vi "Teleop.vi"(10 "Match Info":T1={"Autonomous Elapsed Seconds"=0.0, "TeleOp Elapsed Seconds"=0.0, "Disabled Elapsed Seconds"=0.0, "Visited Autonomous"=FALSE, "Visited TeleOp"=FALSE, "Visited Disabled"=FALSE, "Autonomous Settings"={"Autonomous Style"=enum."Independent", "VI Refnum"=refnum}}, 11 "Call Context":T2) -> ()   [LabVIEW 2013]
doc: "This VI is called for each TeleOp packet received from the DS where the robot is not disabled. It is often used to read from the joysticks and update I/O or to update setpoints for timed control loops. It should complete and return within 20 milliseconds or it may miss DS packets."
uses:
  <vilib>/Rock Robotics/WPI/DriverStation/WPI_DriverStationDerivedRobotMode.ctl
  <vilib>/Rock Robotics/WPI/DriverStation/WPI_DriverStationMatch Info.ctl
  Robot Global Data.vi
  <vilib>/Rock Robotics/WPI/Joystick/WPI_JoystickGetSetRefNum.vi
  <vilib>/Rock Robotics/WPI/RobotDrive/WPI_RobotDriveGetSetRefNum.vi
  <vilib>/Rock Robotics/WPI/RobotDrive/WPI_RobotDriveArcadeDrive_Standard(NoSaturation).vi
panel:
  out "Yaxis 2":dbl
  in  "YAxis":dbl
  in  "StockArcade?":bool
  in  "Ramp?":bool=TRUE
  in  "Yaxis":dbl
  in  "Mult":dbl=0.0010912021824043647
  in  "x":dbl=1.1
  in  "y":dbl=0.95
  out "Numeric 1":dbl(slide) scale=0.0..100.0
  out "Boolean 2":bool
  out "Boolean 1":bool
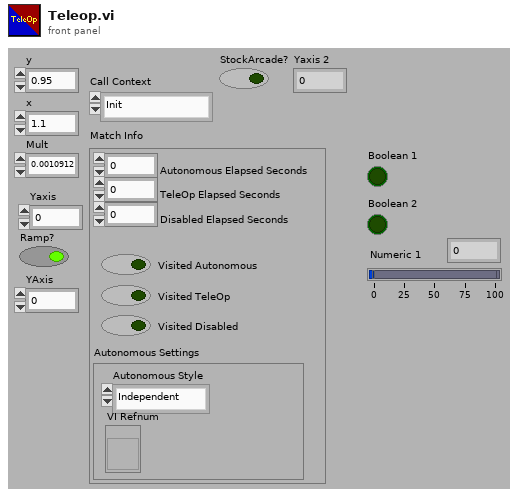
[diagram p1: front panel]
types:
  T1 = typedef "WPI_DriverStationMatch Info.ctl" = cluster{"Autonomous Elapsed Seconds":dbl, "TeleOp Elapsed Seconds":dbl, "Disabled Elapsed Seconds":dbl, "Visited Autonomous":bool, "Visited TeleOp":bool, "Visited Disabled":bool, "Autonomous Settings":cluster{"Autonomous Style":enum16{"Iterative", "Independent"}, "VI Refnum":refnum<vi>}}
  T2 = typedef "WPI_DriverStationDerivedRobotMode.ctl" = enum16{"Init", "Execute", "Stop"}
  T3 = typedef "WPI_JoystickDevRef.ctl" = cluster{"Device":T4}
  T4 = typedef "WPI_JoystickDeviceEnum.ctl" = enum16{"USB 1", "USB 2", "USB 3", "USB 4", "Kinect 1", "Kinect 2"}
  T5 = cluster{"axis 1 (x)":dbl, "axis 2 (y)":dbl, "axis 3 (throttle)":dbl, "axis 4":dbl, "axis 5":dbl, "axis 6":dbl}
  T6 = typedef "WPI_JoystickButtonState.ctl" = cluster{"Button 1":bool, "Button 2":bool, "Button 3":bool, "Button 4":bool, "Button 5":bool, "Button 6":bool, "Button 7":bool, "Button 8":bool, "Button 9":bool, "Button 10":bool, "Button 11":bool, "Button 12":bool}
  T7 = typedef "WPI_MotorControlDeviceRef.ctl" = cluster{"DeviceStatus":errorcluster, "Type":enum16{"PWM", "CAN"}, "PWM":cluster{"Digital Module":T8, "PWM Channel":T9, "DeadBand":T10}, "CAN":cluster{"Device Number":u8, "Control Mode":T11, "Semaphore":T12, "Max Vout":dbl}, "Invert":bool, "TransformRef":T13, "InvTransformRef":T13}
  T8 = typedef "FPGA_TypedefDigitalModule.ctl" = enum16{"Digital Module 1", "Digital Module 2"}
  T9 = typedef "FPGA_DIOPWMChannel.ctl" = enum8{"PWM 1", "PWM 2", "PWM 3", "PWM 4", "PWM 5", "PWM 6", "PWM 7", "PWM 8", "PWM 9", "PWM 10", "Invalid"}
  T10 = typedef "WPI_PWMDeadband.ctl" = cluster{"Name":string, "maxPositivePwm":i32, "minPositivePwm":i32, "centerPwm":i32, "maxNegativePwm":i32, "minNegativePwm":i32, "angularRange":u16}
  T11 = typedef "WPI_CANJaguar_ControlMode.ctl" = enum8{"Percent VBus", "Current", "Speed", "Position", "Voltage"}
  T12 = typedef "Semaphore RefNum" = refnum<k1>
  T13 = typedef "WPI_PWMTransform_ConPane.ctl" = refnum<vi>
  T14 = typedef "WPI_RobotDriveDevRef.ctl" = cluster{"DevStatus":errorcluster, "Motors[]":T7[], "Square Inputs":bool, "Max Output":dbl, "Isochronous":bool}
  T15 = typedef "WPI_ServoDeviceRef.ctl" = cluster{"DeviceStatus":errorcluster, "Digital Module":T8, "PWM Channel":T9, "DeadBand":T10}
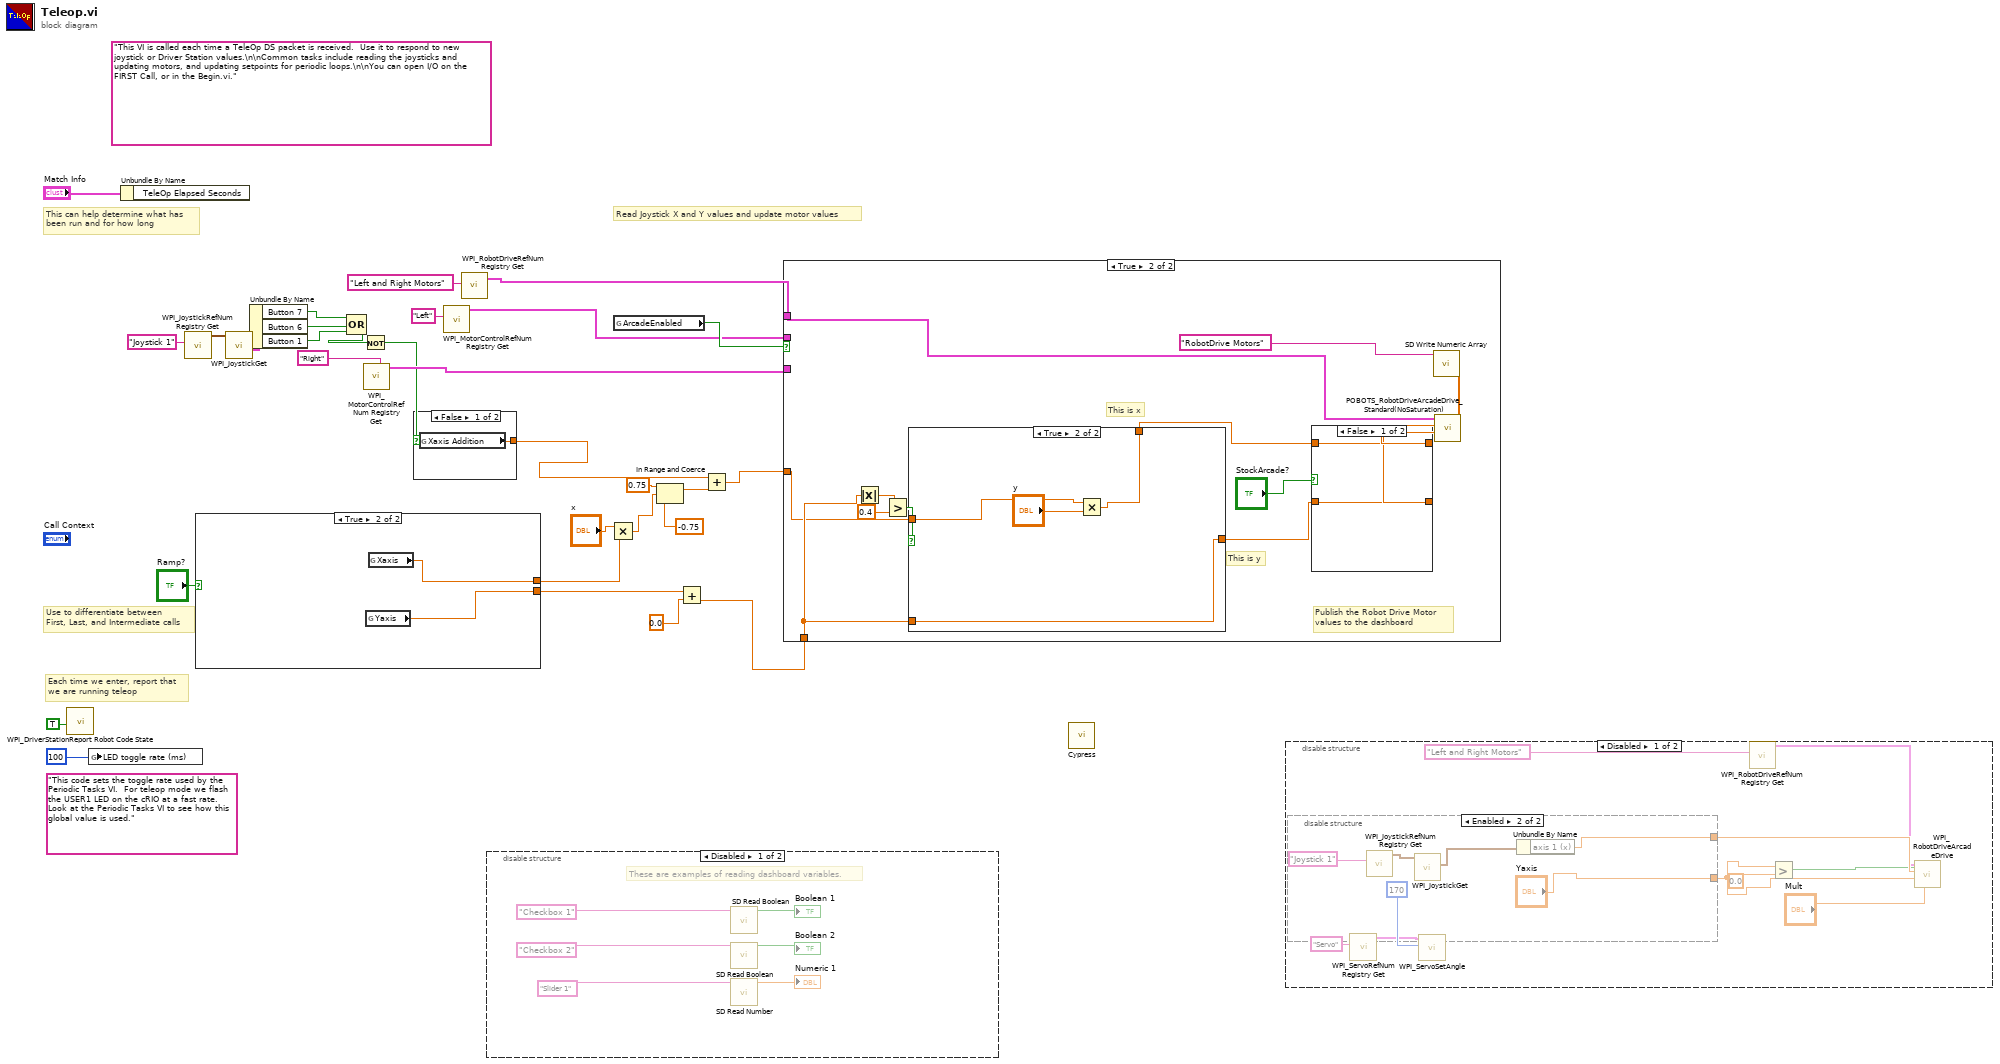
[diagram p0: block diagram]
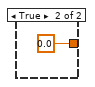
[diagram p2: hidden frame]
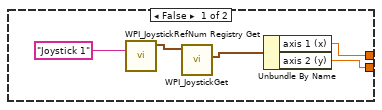
[diagram p3: hidden frame]
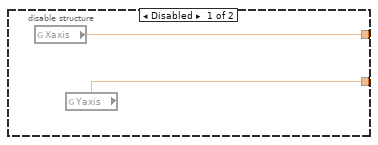
[diagram p4: hidden frame]
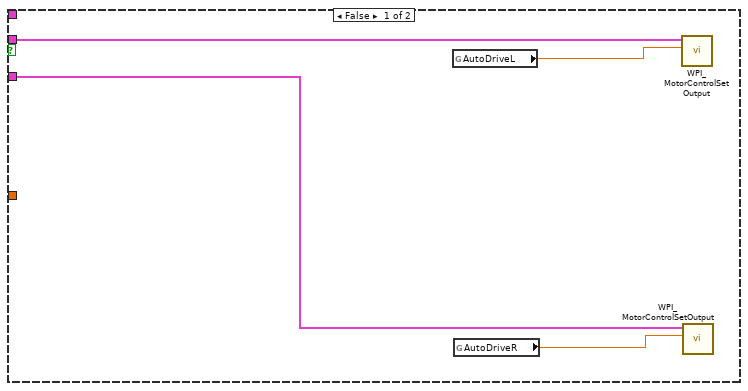
[diagram p6: hidden frame]
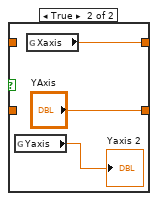
[diagram p7: hidden frame]
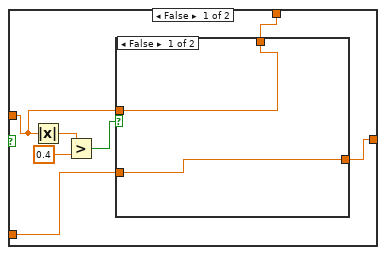
[diagram p8: hidden frame]
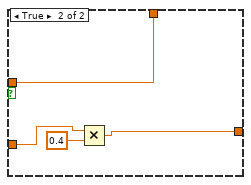
[diagram p9: hidden frame]
diagram:
  (unwired) "This code sets the toggle rate used by the Periodic Tasks VI.  For teleop mode we flash the USER1 LED on the cRIO at a fast rate.  Look at the Periodic Tasks VI to see how this global value is used."
  (unwired) "This VI is called each time a TeleOp DS packet is received.  Use it to respond to new joystick or Driver Station values.\n\nCommon tasks include reading the joysticks and updating motors, and updating setpoints for periodic loops.\n\nYou can open I/O on the FIRST Call, or in the Begin.vi."
  # "Publish the Robot Drive Motor\nvalues to the dashboard"
  # "Read Joystick X and Y values and update motor values"
  # "Each time we enter, report that\nwe are running teleop"
  # "Use to differentiate between\nFirst, Last, and Intermediate calls"
  # "This can help determine what has\nbeen run and for how long"
  n1 = call <vilib>:"WPI_DriverStationReport Robot Code State.vi"("TeleOp"=TRUE ("Autonomous")) -> ()  [unwired: 10 in, 1 out]
  n2 = global write "Robot Global Data.vi" "LED toggle rate (ms)"(u32 100 ("LED ms toggle rate")) -> ()
  n3 = Unbundle By Name("Match Info") -> ()  [unwired: 1 out]
  n4 = call <vilib>:"WPI_JoystickRefNum Registry Get.vi"("refnum name"="Joystick 1") -> ("JoystickDevRef"=w7:T3)  [unwired: 9 in, 1 out]
  n5 = case shown="True" "Ramp?" {
    tunnel: [w32 w37] -> w24
    tunnel: [w31 w36] -> w22
    frame False {
      n6 = call <vilib>:"WPI_JoystickRefNum Registry Get.vi"("refnum name"="Joystick 1") -> ("JoystickDevRef"=w34:T3)  [unwired: 9 in, 1 out]
      n7 = call <vilib>:"WPI_JoystickGet.vi"("JoystickDevRef"=w34) -> ("Axes"=w33:T5)  [unwired: 4 in, 2 out]
      n8 = Unbundle By Name(w33) -> ("axis 1 (x)"=w32:dbl, "axis 2 (y)"=w31:dbl)
    }
    frame True {
      n9 = global read "Robot Global Data.vi" "Yaxis"() -> (w36:dbl)
      n10 = global read "Robot Global Data.vi" "Xaxis"() -> (w37:dbl)
    }
  }
  n11 = call <vilib>:"WPI_JoystickGet.vi"("JoystickDevRef"=w7) -> ("Buttons"=w6:T6)  [unwired: 4 in, 2 out]
  n12 = Unbundle By Name(w6) -> ("Button 7"=w1:bool, "Button 6"=w2:bool, "Button 1"=w5:bool)
  n13 = Compound Arithmetic op=OR(w1, w2, w5) -> (w3:bool)
  n14 = Not(x=w3) -> (.not. x?=w4:bool)
  n15 = call <vilib>:"WPI_MotorControlRefNum Registry Get.vi"("refnum name"="Right") -> ("MotorControlDevRef"=w17:T7)  [unwired: 9 in, 1 out]
  n16 = case shown="False" w4 {
    tunnel: [w38 0.0 ("x")] -> w9
    frame False {
      n17 = global read "Robot Global Data.vi" "Xaxis Addition"() -> (w38:dbl)
    }
    frame True {
    }
  }
  n18 = call <vilib>:"WPI_MotorControlRefNum Registry Get.vi"("refnum name"="Left") -> ("MotorControlDevRef"=w18:T7)  [unwired: 9 in, 1 out]
  n19 = call <vilib>:"WPI_RobotDriveRefNum Registry Get.vi"("refnum name"="Left and Right Motors") -> ("RobotDriveDevRef"=w27:T14)  [unwired: 9 in, 1 out]
  n20 = disable-structure shown="Disabled" {
    frame Disabled {
      # "These are examples of reading dashboard variables."
      n21 = call <vilib>:"SD Read Boolean.vi"("Name"="Checkbox 1" ("refnum name")) -> ("Boolean"=→"Boolean 1":bool)  [unwired: 8 in, 2 out]
      n22 = call <vilib>:"SD Read Boolean.vi"("Name"="Checkbox 2" ("refnum name")) -> ("Boolean"=→"Boolean 2":bool)  [unwired: 8 in, 2 out]
      n23 = call <vilib>:"SD Read Number.vi"("Name"="Slider 1" ("refnum name")) -> ("Numeric"=→"Numeric 1":dbl)  [unwired: 8 in, 2 out]
    }
    frame Enabled {
    }
  }
  n24 = Multiply(x="x", y=w24) -> (x*y=w15:dbl)
  n25 = global read "Robot Global Data.vi" "ArcadeEnabled"() -> (w21:bool)
  n26 = In Range and Coerce(upper limit=0.75, x=w15, lower limit=-0.75) -> (coerced(x)=w14:dbl)  [unwired: 1 out]
  n27 = Add(x=w22, y=0.0) -> (x+y=w23:dbl)
  n28 = Add(x=w9, y=w14) -> (x+y=w25:dbl)
  n29 = case shown="True" w21 {
    tunnel: w27 -> [_ w62]
    tunnel: w25 -> [_ w55]
    tunnel: w23 -> [_ w57]
    tunnel: w18 -> [w49 _]
    tunnel: w17 -> [w48 _]
    frame False {
      n30 = global read "Robot Global Data.vi" "AutoDriveL"() -> (w47:dbl)
      n31 = global read "Robot Global Data.vi" "AutoDriveR"() -> (w46:dbl)
      n32 = call <vilib>:"WPI_MotorControlSetOutput.vi"("Output"=w47, "MotorControlDevRef"=w49) -> ()  [unwired: 7 in, 3 out]
      n33 = call <vilib>:"WPI_MotorControlSetOutput.vi"("Output"=w46, "MotorControlDevRef"=w48) -> ()  [unwired: 7 in, 3 out]
    }
    frame True {
      # "This is y"
      # "This is x"
      n34 = Absolute Value(x=w57) -> (abs(x)=w58:dbl)
      n35 = Greater?(x=w58, y=0.4) -> (0:w59:bool)
      n36 = case shown="True" w59 {
        tunnel: w57 -> [w68 w84]
        tunnel: [w69 w84] -> w50
        tunnel: [w71 w81] -> w51
        tunnel: w55 -> [w70 w82]
        frame False {
          n37 = Absolute Value(x=w70) -> (abs(x)=w74:dbl)
          n38 = Greater?(x=w74, y=0.4) -> (0:w73:bool)
          n39 = case shown="False" w73 {
            tunnel: [w75 w80] -> w71
            tunnel: w70 -> [w75 w80]
            tunnel: [w76 w79] -> w69
            tunnel: w68 -> [w76 w77]
            frame False {
            }
            frame True {
              n40 = Multiply(x=w77, y=0.4) -> (x*y=w79:dbl)
            }
          }
        }
        frame True {
          n41 = Multiply(x=w82, y="y") -> (x*y=w81:dbl)
        }
      }
      n42 = case shown="False" "StockArcade?" {
        tunnel: [w64 w67] -> w54
        tunnel: [w63 "YAxis"] -> w53
        tunnel: w51 -> [w64 _]
        tunnel: w50 -> [w63 _]
        frame False {
        }
        frame True {
          n43 = global read "Robot Global Data.vi" "Yaxis"() -> (→"Yaxis 2":dbl)
          n44 = global read "Robot Global Data.vi" "Xaxis"() -> (w67:dbl)
        }
      }
      n45 = call "POBOTS_RobotDriveArcadeDrive_Standard(NoSaturation).vi"("Y axis value"=w53, "X axis value"=w54, "RobotDriveDevRef"=w62) -> ("Motor Values"=w60:dbl[])  [unwired: 3 in, 5 out]
      n46 = call <vilib>:"SD Write Numeric Array.vi"("Numeric Array"=w60, "Name"="RobotDrive Motors") -> ()  [unwired: 8 in, 2 out]
    }
  }
  n47 = call "Cypress.vi"() -> ()  [unwired: 12 in]
  n48 = disable-structure shown="Disabled" {
    frame Disabled {
      n49 = disable-structure shown="Enabled" {
        disable-tunnel: [w96 w98] -> w94
        disable-tunnel: [w95 "Yaxis"] -> w90
        frame Disabled {
          n50 = global read "Robot Global Data.vi" "Xaxis"() -> (w96:dbl)
          n51 = global read "Robot Global Data.vi" "Yaxis"() -> (w95:dbl)
        }
        frame Enabled {
          n52 = call <vilib>:"WPI_JoystickRefNum Registry Get.vi"("refnum name"="Joystick 1") -> ("JoystickDevRef"=w100:T3)  [unwired: 9 in, 1 out]
          n53 = call <vilib>:"WPI_JoystickGet.vi"("JoystickDevRef"=w100) -> ("Axes"=w99:T5)  [unwired: 4 in, 2 out]
          n54 = Unbundle By Name(w99) -> ("axis 1 (x)"=w98:dbl)
        }
      }
      n55 = call <vilib>:"WPI_ServoRefNum Registry Get.vi"("refnum name"="Servo") -> ("ServoDeviceRef"=w85:T15)  [unwired: 9 in, 1 out]
      n56 = call <vilib>:"WPI_ServoSetAngle.vi"("Angle"=170, "ServoDeviceRef"=w85) -> ()  [unwired: 8 in, 2 out]
      n57 = call <vilib>:"WPI_RobotDriveRefNum Registry Get.vi"("refnum name"="Left and Right Motors") -> ("RobotDriveDevRef"=w92:T14)  [unwired: 9 in, 1 out]
      n58 = Greater?(x=w90, y=0.0 ("x")) -> (0:w89:bool)
      n59 = call-poly <vilib>:"WPI_RobotDriveArcadeDrive.vi"(6:"Mult", 7:w89, "Y axis value"=w90, "X axis value"=w94, "RobotDriveDevRef"=w92) -> ()  [unwired: 4 in, 3 out]
    }
    frame Enabled {
    }
  }
